vi "Get Group Status.vi"(4 "error in (no error)":errorcluster, 6 "Group Number (1)":i32=1 min=1, 7 "VISA resource name":refnum<visa-resource-name>) -> (0 "error out":errorcluster, 2 "Group Status (F:group power is OFF)":bool, 3 "VISA resource name out":refnum<visa-resource-name>)   [LabVIEW 2018, in "Newport ESP301.lvlib"]
doc: "This command (HO) turns power ON of all axes assigned to a group. Refer MO command to turn the power ON of individual axes. The group power is assumed to be ON if power to all axes in the group is ON."
uses:
  Newport ESP301.lvlib
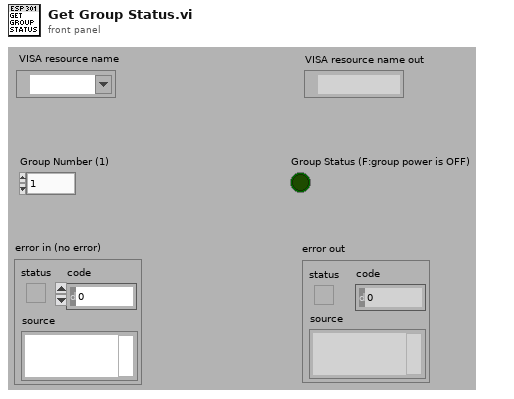
[diagram p1: front panel]
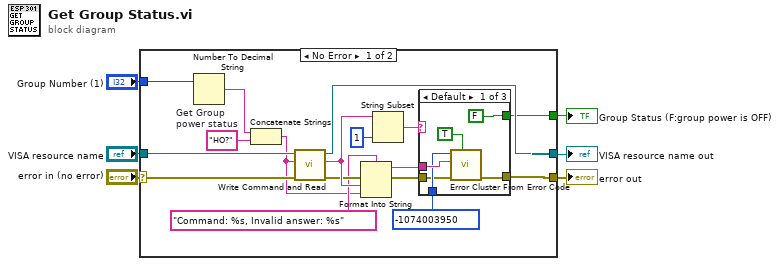
[diagram p0: block diagram]
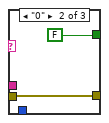
[diagram p2: hidden frame]
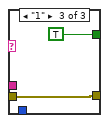
[diagram p3: hidden frame]
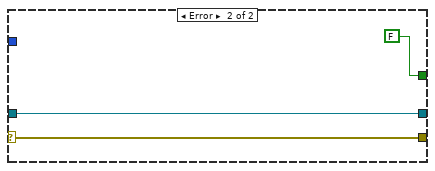
[diagram p4: hidden frame]
diagram:
  n1 = case shown="No Error" "error in (no error)" {
    selector: "error in (no error)" -> [w21 w36]
    tunnel: [w7 w36] -> w6
    tunnel: "VISA resource name" -> [w23 w35]
    tunnel: [w22 w35] -> w5
    tunnel: "Group Number (1)" -> [w18 _]
    tunnel: [w11 FALSE ("Motion Done")] -> w1
    frame No Error {
      w20 = "HO?"  # Get Group  power status
      n2 = Number To Decimal String(number=w18) -> (decimal integer string=w19:string)  [unwired: 1 in]
      n3 = Concatenate Strings(w19, w20) -> (w9:string)
      n4 = call "Write Command and Read.vi"("error in (no error)"=w21, "Command"=w9, "VISA resource name"=w23) -> ("error out"=w12:errorcluster, "Returned string"=w13:string, "VISA resource name out"=w22:refnum<visa-resource-name>)  [unwired: 4 in]
      n5 = Format Into String(format string="Command: %s, Invalid answer: %s" ("error message (\"\")"), error in=w12, w13, w9) -> (resulting string=w15:string, error out=w8:errorcluster)  [unwired: 1 in]
      n6 = String Subset(string=w13, length (rest)=1 ("longueur (reste)")) -> (substring=w16:string)  [unwired: 1 in]
      n7 = case shown="Default" w16 {
        tunnel: [FALSE ("Motion Done") FALSE ("Motion Done") TRUE ("Motion Done")] -> w11
        tunnel: w15 -> [w27 _ _]
        tunnel: -1074003950 ("error code (0)") -> [w26 _ _]
        tunnel: w8 -> [w25 w30 w32]
        tunnel: [w24 w30 w32] -> w7
        frame Default {
          n8 = call <vilib>:"Error Cluster From Error Code.vi"("show call chain? (False)"=TRUE, "error in (no error)"=w25, "error message (\"\")"=w27, "error code (0)"=w26) -> ("error out"=w24:errorcluster)  [unwired: 5 in]
        }
        frame "0" {
        }
        frame "1" {
        }
      }
    }
    frame Error {
    }
  }
  "error out" <- w6
  "VISA resource name out" <- w5
  "Group Status (F:group power is OFF)" <- w1
